vi "Read Value.vi"(8 "error in (no error)":errorcluster, 11 "int32 in":refnum<class "sint64.lvclass">) -> (0 "error out":errorcluster, 2 "Value":i64, 3 "int32 out":refnum<class "sint64.lvclass">)   [LabVIEW 2020, in "Protobuf RAW.lvlib" / "sint64.lvclass"]
uses:
  sint64.lvclass
  sint64.lvclass/sint64.ctl
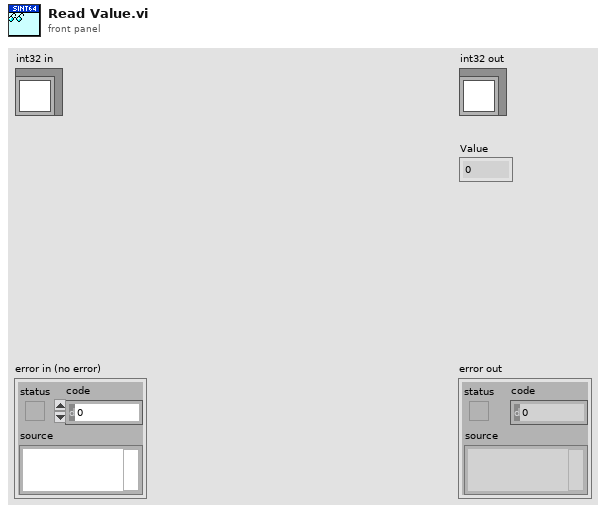
[diagram p1: front panel]
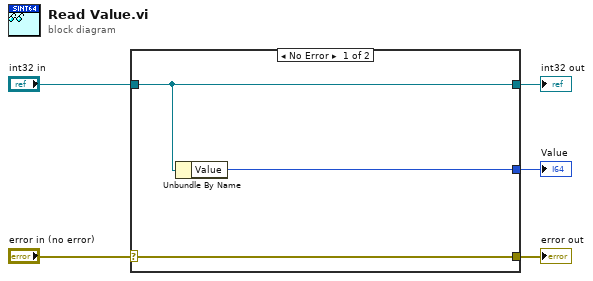
[diagram p0: block diagram]
diagram:
  n1 = case shown="No Error" "error in (no error)" {
    selector: "error in (no error)" -> [w8 w9]
    tunnel: [w8 w9] -> w4
    tunnel: [w7 w10] -> w2
    tunnel: "int32 in" -> [w7 w10]
    tunnel: [w6 _] -> w1
    frame No Error {
      n2 = Unbundle By Name(w7) -> ("Value"=w6:i64)
    }
    frame Error {
    }
  }
  "error out" <- w4
  "int32 out" <- w2
  "Value" <- w1
